vi "Drive Encoder Test.vi"   [LabVIEW 2014]
uses:
  <vilib>/Rock Robotics/WPI/DriverStation/WPI_DriverStationRobotMode2.ctl
  Begin/Global Variables.vi
  Begin/Global RefNums.vi
  Begin/Global Constants.vi
  <vilib>/Utility/file.llb/Write To Spreadsheet File (DBL).vi
types:
  T1 = typedef "WPI_DriverStationRobotMode2.ctl" = enum16{"Autonomous Disabled", "Autonomous Enabled", "Teleop Disabled", "Teleop Enabled", "Disconnected", "Finish", "Test Disabled", "Test Enabled", "Emergency Stopped"}
  T2 = typedef "WPI_AnalogChannelDevRef.ctl" = cluster{"DevStatus":errorcluster, "Controller":T3, "Analog Channel":T4}
  T3 = typedef "FPGA_TypedefAnalogModule.ctl" = enum16{"Controller 1"}
  T4 = typedef "FPGA_AIChannel.ctl" = enum8{"AI 0", "AI 1", "AI 2", "AI 3", "AI MXP 0", "AI MXP 1", "AI MXP 2", "AI MXP 3", "Invalid"}
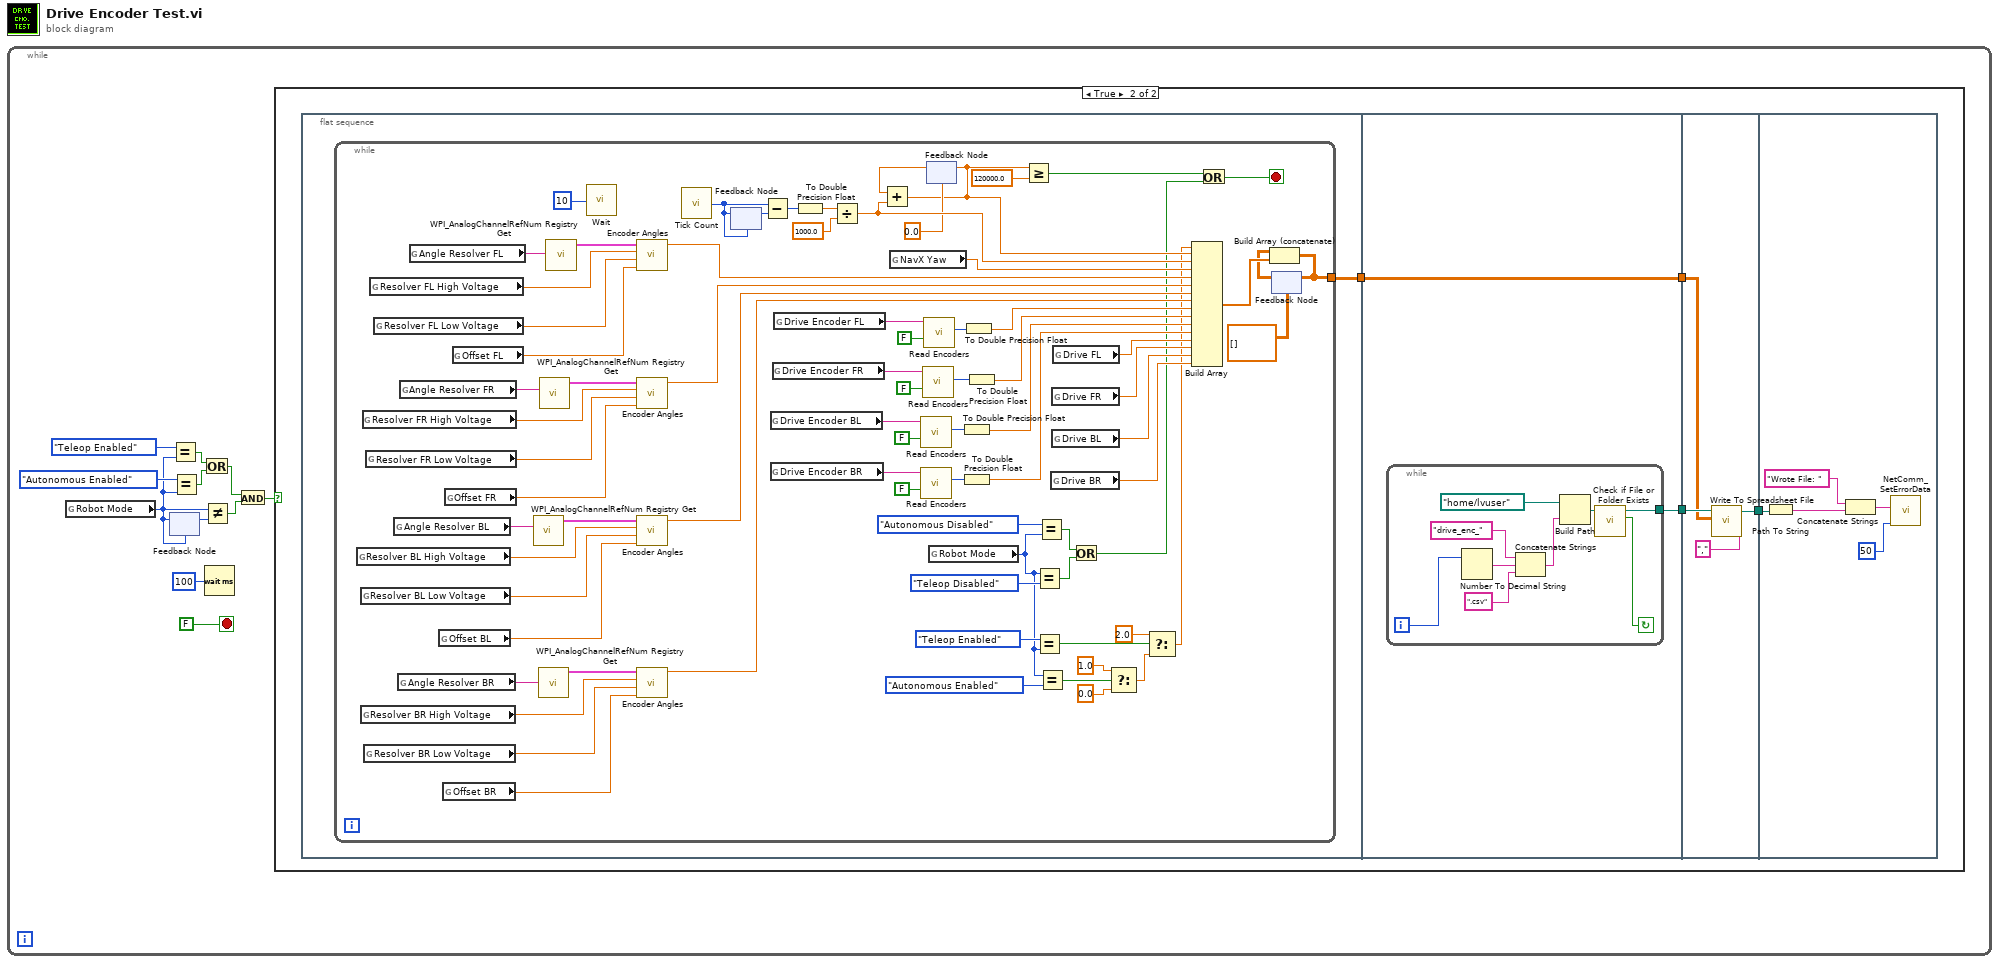
[diagram p0: block diagram]
diagram:
  n1 = while {
    stop <- FALSE stop-if-true
    n2 = global read "Global Variables.vi" "Robot Mode"() -> (w4:T1)
    n3 = feedback-in #1(w4) -> ()
    n4 = feedback #1(w4) -> (w9:T1)
    n5 = Equal?(x=WPI_DriverStationRobotMode2."Teleop Enabled", y=w4) -> (x = y?=w3:bool)
    n6 = Equal?(x=WPI_DriverStationRobotMode2."Autonomous Enabled", y=w4) -> (x = y?=w2:bool)
    n7 = Or(x=w3, y=w2) -> (x .or. y?=w1:bool)
    n8 = Not Equal?(x=w4, y=w9) -> (x != y?=w8:bool)
    n9 = Wait (ms)(milliseconds to wait=u32 100) -> ()  [unwired: 1 out]
    n10 = And(x=w1, y=w8) -> (x .and. y?=w7:bool)
    n11 = case shown="True" w7 {
      frame False {
      }
      frame True {
        n12 = flat-sequence {
          tunnel: [w16] -> w15
          tunnel: w15 -> [w94]
          tunnel: [w95] -> w14
          tunnel: [w94] -> w13
          tunnel: w14 -> [w107]
          tunnel: w13 -> [w106]
          tunnel: [w105] -> w12
          tunnel: w12 -> [w109]
          frame #0 {
            n13 = while {
              tunnel: [w53] -> w16
              stop <- w29 stop-if-true
              n14 = global read "Global Constants.vi" "Resolver BL High Voltage"() -> (w79:dbl)
              n15 = global read "Global Constants.vi" "Resolver BL Low Voltage"() -> (w78:dbl)
              n16 = global read "Global Constants.vi" "Resolver BR High Voltage"() -> (w81:dbl)
              n17 = global read "Global Constants.vi" "Resolver FR High Voltage"() -> (w85:dbl)
              n18 = global read "Global Constants.vi" "Resolver BR Low Voltage"() -> (w80:dbl)
              n19 = global read "Global Constants.vi" "Resolver FR Low Voltage"() -> (w84:dbl)
              n20 = global read "Global Constants.vi" "Resolver FL High Voltage"() -> (w83:dbl)
              n21 = global read "Global Constants.vi" "Resolver FL Low Voltage"() -> (w82:dbl)
              n22 = global read "Global RefNums.vi" "Angle Resolver BL"() -> (w92:string)
              n23 = global read "Global RefNums.vi" "Angle Resolver BR"() -> (w91:string)
              n24 = global read "Global RefNums.vi" "Angle Resolver FR"() -> (w93:string)
              n25 = global read "Global RefNums.vi" "Angle Resolver FL"() -> (w90:string)
              n26 = global read "Global Constants.vi" "Offset BL"() -> (w74:dbl)
              n27 = global read "Global Constants.vi" "Offset BR"() -> (w75:dbl)
              n28 = global read "Global Constants.vi" "Offset FR"() -> (w77:dbl)
              n29 = global read "Global Constants.vi" "Offset FL"() -> (w76:dbl)
              n30 = call <vilib>:"WPI_AnalogChannelRefNum Registry Get.vi"("refnum name"=w92) -> ("AIDeviceRef"=w86:T2)  [unwired: 9 in, 1 out]
              n31 = call <vilib>:"WPI_AnalogChannelRefNum Registry Get.vi"("refnum name"=w91) -> ("AIDeviceRef"=w87:T2)  [unwired: 9 in, 1 out]
              n32 = call <vilib>:"WPI_AnalogChannelRefNum Registry Get.vi"("refnum name"=w93) -> ("AIDeviceRef"=w89:T2)  [unwired: 9 in, 1 out]
              n33 = call <vilib>:"WPI_AnalogChannelRefNum Registry Get.vi"("refnum name"=w90) -> ("AIDeviceRef"=w88:T2)  [unwired: 9 in, 1 out]
              n34 = call "Wait"("Count(mSec)"=u32 10) -> ()  [unwired: 1 out]
              n35 = call "Encoder Angles.vi"("calibration angle"=w76, "low voltage"=w82, "top voltage"=w83, "AIDeviceRef Encoder"=w88) -> ("encoder angle"=w45:dbl)  [unwired: 7 in]
              n36 = call "Encoder Angles.vi"("calibration angle"=w77, "low voltage"=w84, "top voltage"=w85, "AIDeviceRef Encoder"=w89) -> ("encoder angle"=w44:dbl)  [unwired: 7 in]
              n37 = call "Encoder Angles.vi"("calibration angle"=w74, "low voltage"=w78, "top voltage"=w79, "AIDeviceRef Encoder"=w86) -> ("encoder angle"=w43:dbl)  [unwired: 7 in]
              n38 = call "Encoder Angles.vi"("calibration angle"=w75, "low voltage"=w80, "top voltage"=w81, "AIDeviceRef Encoder"=w87) -> ("encoder angle"=w42:dbl)  [unwired: 7 in]
              n39 = call "Tick Count"() -> ("Tick Count(uSec)"=w60:u32)
              n40 = feedback-in #2(w60) -> ()
              n41 = feedback #2(w60) -> (w59:u32)
              n42 = Subtract(x=w60, y=w59) -> (x-y=w51:u32)
              n43 = global read "Global RefNums.vi" "Drive Encoder BL"() -> (w73:string)
              n44 = global read "Global RefNums.vi" "Drive Encoder BR"() -> (w70:string)
              n45 = global read "Global RefNums.vi" "Drive Encoder FR"() -> (w68:string)
              n46 = global read "Global RefNums.vi" "Drive Encoder FL"() -> (w69:string)
              n47 = To Double Precision Float(number=w51) -> (double precision float=w58:dbl)
              n48 = Divide(x=w58, y=1000.0) -> (x/y=w50:dbl)
              n49 = global read "Global Variables.vi" "NavX Yaw"() -> (w61:dbl)
              n50 = call "Read Encoders.vi"("Reset Encoders"=FALSE, "Encoder"=w73) -> ("Counts"=w65:i32)  [unwired: 9 in]
              n51 = call "Read Encoders.vi"("Reset Encoders"=FALSE, "Encoder"=w70) -> ("Counts"=w62:i32)  [unwired: 9 in]
              n52 = call "Read Encoders.vi"("Reset Encoders"=FALSE, "Encoder"=w68) -> ("Counts"=w64:i32)  [unwired: 9 in]
              n53 = call "Read Encoders.vi"("Reset Encoders"=FALSE, "Encoder"=w69) -> ("Counts"=w63:i32)  [unwired: 9 in]
              n54 = feedback #3(0.0) -> (w49:dbl)
              n55 = Add(x=w49, y=w50) -> (x+y=w46:dbl)
              n56 = feedback-in #3(w46) -> ()
              n57 = global read "Global Variables.vi" "Robot Mode"() -> (w23:T1)
              n58 = To Double Precision Float(number=w65) -> (double precision float=w39:dbl)
              n59 = To Double Precision Float(number=w62) -> (double precision float=w38:dbl)
              n60 = To Double Precision Float(number=w63) -> (double precision float=w41:dbl)
              n61 = To Double Precision Float(number=w64) -> (double precision float=w40:dbl)
              n62 = Greater Or Equal?(x=w46, y=120000.0) -> (x >= y?=w28:bool)
              n63 = Equal?(x=w23, y=WPI_DriverStationRobotMode2."Teleop Disabled" ("x")) -> (x = y?=w31:bool)
              n64 = Equal?(x=WPI_DriverStationRobotMode2."Teleop Enabled", y=w23) -> (x = y?=w25:bool)
              n65 = Equal?(x=WPI_DriverStationRobotMode2."Autonomous Disabled", y=w23) -> (x = y?=w30:bool)
              n66 = Equal?(x=w23, y=WPI_DriverStationRobotMode2."Autonomous Enabled" ("x")) -> (x = y?=w22:bool)
              n67 = global read "Global Variables.vi" "Drive BR"() -> (w34:dbl)
              n68 = global read "Global Variables.vi" "Drive FR"() -> (w36:dbl)
              n69 = global read "Global Variables.vi" "Drive BL"() -> (w35:dbl)
              n70 = global read "Global Variables.vi" "Drive FL"() -> (w37:dbl)
              n71 = Or(x=w30, y=w31) -> (x .or. y?=w27:bool)
              n72 = Select(t=1.0, s=w22, f=0.0) -> (s? t:f=w21:dbl)
              n73 = Select(t=2.0, s=w25, f=w21) -> (s? t:f=w17:dbl)
              n74 = Build Array(w17, w46, w50, w61, w45, w44, w43, w42, w41, w40, w39, w38, w37, w36, w35, w34) -> (w56:dbl[])
              n75 = Or(x=w28, y=w27) -> (x .or. y?=w29:bool)
              n76 = feedback #4(dbl[][] []) -> (w55:dbl[][])
              n77 = Build Array (concatenate)(w55, w56) -> (w53:dbl[][])
              n78 = feedback-in #4(w53) -> ()
            }
          }
          frame #1 {
            n79 = while {
              tunnel: [w97] -> w95
              i -> [w96]
              stop <- w104 continue-if-true
              n80 = Number To Decimal String(number=w96) -> (decimal integer string=w101:string)  [unwired: 1 in]
              n81 = Concatenate Strings("drive_enc_", w101, ".csv") -> (w100:string)
              n82 = Build Path(base path=path "/home/lvuser" ("file path (dialog if empty)"), name or relative path=w100) -> (appended path=w103:path)
              n83 = call <vilib>:"Check if File or Folder Exists.vi"("path"=w103) -> ("file or folder exists?"=w104:bool, "dup path"=w97:path)  [unwired: 8 in, 1 out]
            }
          }
          frame #2 {
            n84 = call-poly <vilib>:"Write To Spreadsheet File.vi"("delimiter (\\t)"="," ("delimiter (\\t)"), "2D data"=w106, "file path (dialog if empty)"=w107) -> ("new file path (Not A Path if cancelled)"=w105:path)  [unwired: 5 in]
          }
          frame #3 {
            n85 = Path To String(path=w109) -> (string=w113:string)
            n86 = Concatenate Strings("Wrote File: ", w113) -> (w111:string)
            n87 = call <vilib>:"NetComm_SetErrorData.vi"("Timeout (ms)"=50, "Error Data"=w111) -> ()  [unwired: 2 in, 8 out]
          }
        }
      }
    }
  }
